vi "SL_Facade.vi"(0 "Data In":T5, 2 "Display State In":T3, 3 "Container State":T4) -> (6 "Data Out":T5, 7 "Display State Out":T3, 8 "Action":T2)   [LabVIEW 2019, in "SL_XControl.xctl"]
uses:
  SL_XControl.xctl
  SL_Data.ctl
  <vilib>/_xctls/Container State.ctl
  SL_State.ctl
  <vilib>/_xctls/Action.ctl
  <vilib>/_xctls/XControlSupport.lvlib
panel:
  out "Toggle":bool
  out "info":string
  in  "Refresh":bool
  in  "Login":bool
  in  "Edit":bool
  in  "Tag":T1
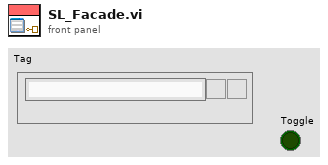
[diagram p1: front panel]
types:
  T1 = cluster{"Property":string, "Type":string, "Data":string}
  T2 = typedef "XControlSupport.lvlib/Action.ctl" = cluster{"Data Changed?":bool, "State Changed?":bool, "Action Name":string}
  T3 = typedef "SL_XControl.xctl/SL_State.ctl" = cluster{"Numeric":dbl}
  T4 = typedef "XControlSupport.lvlib/Container State.ctl" = cluster{"Indicator?":bool, "Run Mode?":bool, " Refnum":refnum<vi>}
  T5 = typedef "SL_XControl.xctl/SL_Data.ctl" = cluster{"Tag":string, "Type":string, "Data":string}
  T6 = enum8{"Enabled", "Disabled", "Disabled and Grayed Out"}
  T7 = cluster{"Name":string, "BaseURL":string, "AppKey":string, "Headers":string[], "Timeout":i32}
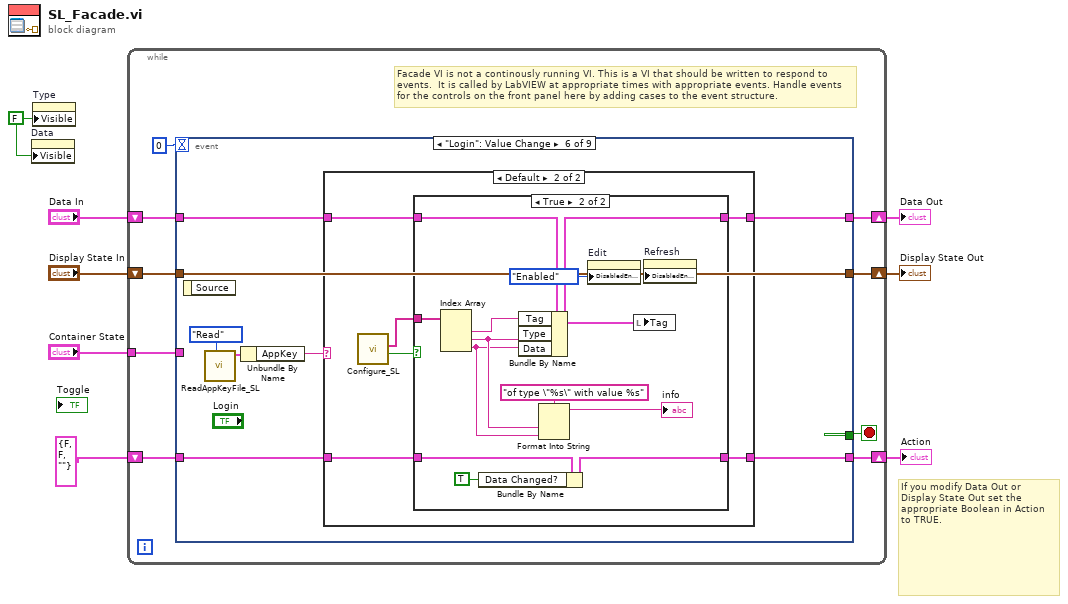
[diagram p0: block diagram]
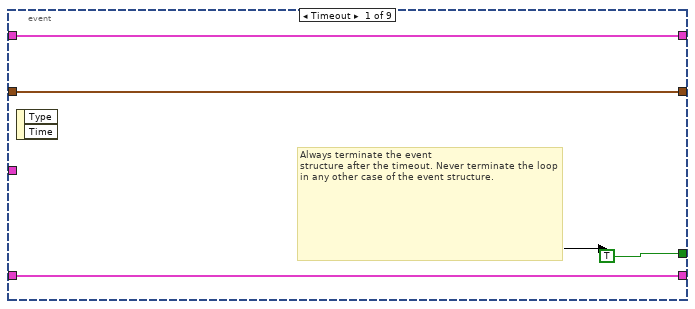
[diagram p2: hidden frame]
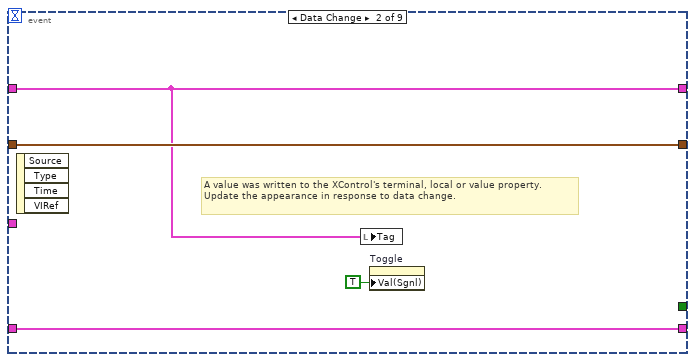
[diagram p3: hidden frame]
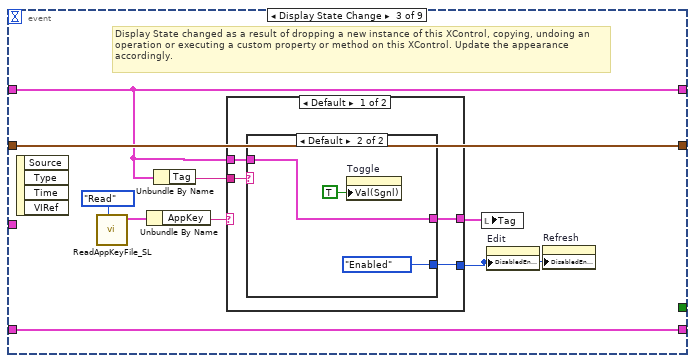
[diagram p4: hidden frame]
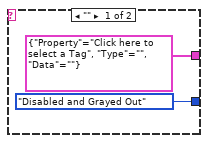
[diagram p5: hidden frame]
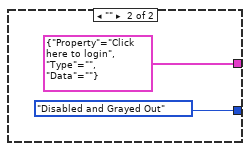
[diagram p6: hidden frame]
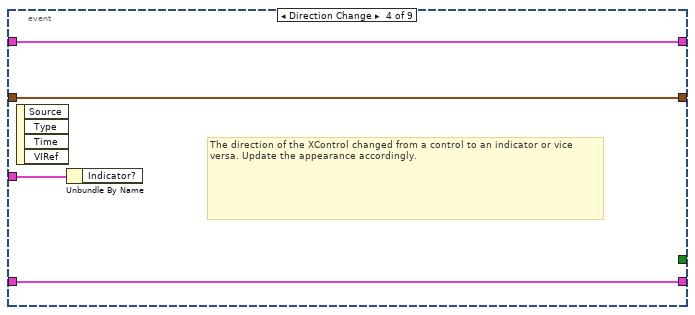
[diagram p7: hidden frame]
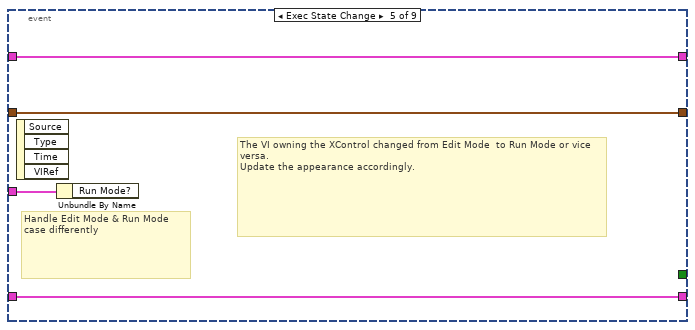
[diagram p8: hidden frame]
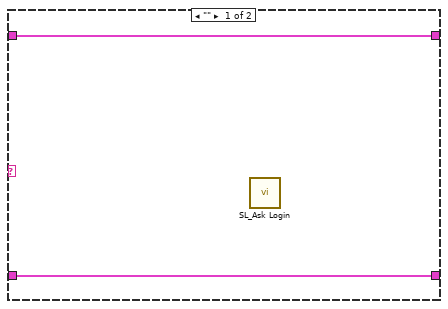
[diagram p9: hidden frame]
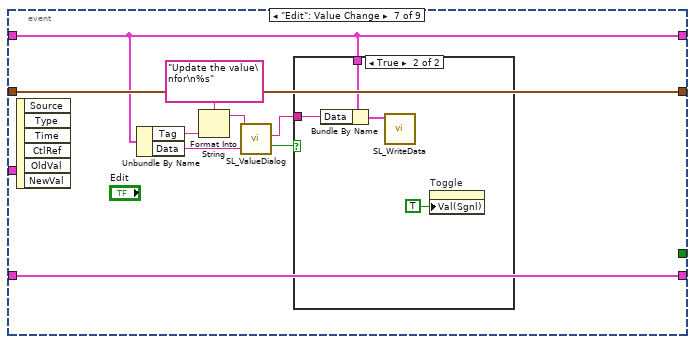
[diagram p11: hidden frame]
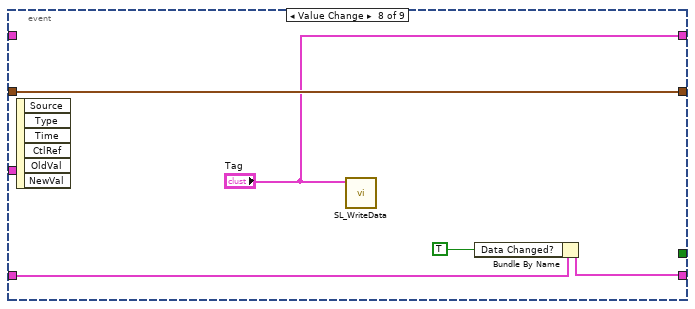
[diagram p13: hidden frame]
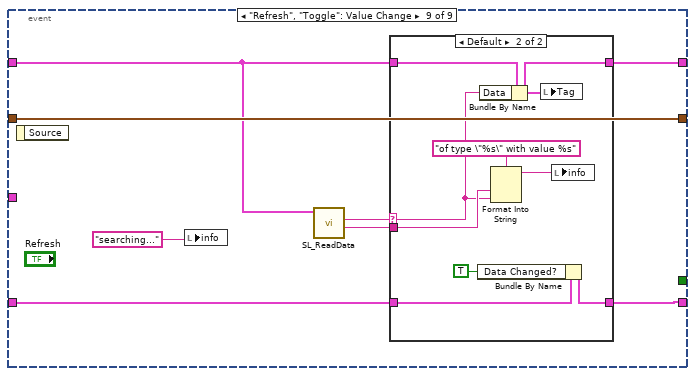
[diagram p14: hidden frame]
diagram:
  w1 = FALSE ("Visible")
  # "If you modify Data Out or\nDisplay State Out set the\nappropriate Boolean in Action\nto TRUE."
  n1 = property on="Data" class="Str"("Visible"=w1) -> ()  [unwired: 2 in, 2 out]
  n2 = property on="Type" class="Str"("Visible"=w1) -> ()  [unwired: 2 in, 2 out]
  n3 = while {
    shift-right: [w16] -> w5
    shift-left: "Display State In" -> [w17]
    tunnel: "Container State" -> [w13]
    shift-right: [w11] -> w8
    shift-left: "Data In" -> [w12]
    shift-right: [w9] -> w3
    shift-left: T2 {"Data Changed?"=FALSE, "State Changed?"=FALSE, "Action Name"=""} ("Action") -> [w10]
    stop <- w15 stop-if-true
    # "Facade VI is not a continously running VI. This is a VI that should be written to respond to events.  It is called by LabVIEW at appropriate times with appropriate events. Handle events for the controls on the front panel here by adding cases to the event structure."
    n4 = event shown="[5] \"Login\": Value Change" {
      selector: _ -> [_ _ _ _ _ _ _ _ _]
      dyn-events: _ -> [_ _ _ _ _ _ _ _ _]
      timeout: 0 -> [_ _ _ _ _ _ _ _ _]
      tunnel: w17 -> [w19 w25 w34 w48 w52 w61 w92 w101 w109]
      tunnel: [w19 w25 w34 w48 w52 w61 w92 w101 w109] -> w16
      tunnel: [TRUE _ _ _ _ _ _ _ _] -> w15
      tunnel: w13 -> [_ _ _ w49 w53 _ _ _ _]
      tunnel: w12 -> [w18 w22 w26 w47 w51 w58 w88 _ w105]
      tunnel: [w18 w22 w26 w47 w51 w57 w88 "Tag" w108] -> w11
      tunnel: [w20 w24 w33 w46 w50 w59 w91 w98 w106] -> w9
      tunnel: w10 -> [w20 w24 w33 w46 w50 w60 w91 w99 w107]
      event Timeout {
        # "Always terminate the event\nstructure after the timeout. Never terminate the loop in any other case of the event structure."
        n5 = event-data() -> ()  [unwired: 1 in, 2 out]
      }
      event Data Change {
        # "A value was written to the XControl's terminal, local or value property.\nUpdate the appearance in response to data change."
        n6 = event-data() -> ()  [unwired: 1 in, 4 out]
        n7 = local write "Tag"(w22) -> ()
        n8 = property on="Toggle" class="Bool (strict)"("Val(Sgnl)"=TRUE ("Value (Signaling)")) -> ()  [unwired: 2 in, 2 out]
      }
      event Display State Change {
        # "Display State changed as a result of dropping a new instance of this XControl, copying, undoing an operation or executing a custom property or method on this XControl. Update the appearance accordingly."
        n9 = event-data() -> ()  [unwired: 1 in, 4 out]
        n10 = call "ReadAppKeyFile_SL.vi"("Task"=enum16{"Read", "Write"}."Read") -> ("Device Out"=w32:T7)  [unwired: 8 in, 2 out]
        n11 = Unbundle By Name(w32) -> ("AppKey"=w31:string)
        n12 = Unbundle By Name(w26) -> ("Tag"=w27:string)
        n13 = case shown="Default" w31 {
          tunnel: [w38 T1 {"Property"="Click here to login", "Type"="", "Data"=""} ("Tag")] -> w30
          tunnel: [w37 T6."Disabled and Grayed Out" ("Disabled")] -> w29
          tunnel: w27 -> [w36 _]
          tunnel: w26 -> [w35 _]
          frame Default {
            n14 = case shown="Default" w36 {
              tunnel: [T1 {"Property"="Click here to select a Tag", "Type"="", "Data"=""} ("Tag") w42] -> w38
              tunnel: [T6."Disabled and Grayed Out" ("Disabled") T6."Enabled" ("Disabled")] -> w37
              tunnel: w35 -> [_ w42]
              frame "" {
              }
              frame Default {
                n15 = property on="Toggle" class="Bool (strict)"("Val(Sgnl)"=TRUE ("Value (Signaling)")) -> ()  [unwired: 2 in, 2 out]
              }
            }
          }
          frame "" {
          }
        }
        n16 = local write "Tag"(w30) -> ()
        n17 = property on="Edit" class="Bool"("DisabledEnum"=w29) -> ()  [unwired: 2 in, 2 out]
        n18 = property on="Refresh" class="Bool"("DisabledEnum"=w29) -> ()  [unwired: 2 in, 2 out]
      }
      event Direction Change {
        # "The direction of the XControl changed from a control to an indicator or vice versa. Update the appearance accordingly."
        n19 = event-data() -> ()  [unwired: 1 in, 4 out]
        n20 = Unbundle By Name(w49) -> ()  [unwired: 1 out]
      }
      event Exec State Change {
        # "The VI owning the XControl changed from Edit Mode  to Run Mode or vice versa.\nUpdate the appearance accordingly."
        # "Handle Edit Mode & Run Mode\ncase differently"
        n21 = event-data() -> ()  [unwired: 1 in, 4 out]
        n22 = Unbundle By Name(w53) -> ()  [unwired: 1 out]
      }
      event "Login": Value Change {
        n23 = event-data() -> ()  [unwired: 1 in, 1 out]
        n24 = call "ReadAppKeyFile_SL.vi"("Task"=enum16{"Read", "Write"}."Read") -> ("Device Out"=w56:T7)  [unwired: 8 in, 2 out]
        n25 = Unbundle By Name(w56) -> ("AppKey"=w54:string)
        n26 = case shown="Default" w54 {
          tunnel: w60 -> [w62 w69]
          tunnel: [w62 w68] -> w59
          tunnel: w58 -> [w63 w67]
          tunnel: [w63 w66] -> w57
          frame "" {
            n27 = call "SL_Ask Login.vi"() -> ()  [unwired: 10 in, 2 out]
          }
          frame Default {
            n28 = call "Configure_SL.vi"() -> ("changed?"=w65:bool, "Property"=w64:string[])  [unwired: 10 in]
            n29 = case shown="True" w65 {
              tunnel: w67 -> [w71 w83]
              tunnel: [w71 w78] -> w66
              tunnel: w64 -> [_ w82]
              tunnel: w69 -> [w70 w80]
              tunnel: [w70 w79] -> w68
              frame False {
              }
              frame True {
                w73 = T6."Enabled" ("Disabled")
                n30 = Index Array(array=w82) -> (element #1=w72:string, element #2=w76:string, element #3=w75:string)  [unwired: 3 in]
                n31 = Bundle By Name(cluster=w80, "Data Changed?"=TRUE) -> (w79:T2)
                n32 = Bundle By Name(cluster=w83, "Tag"=w72, "Type"=w76, "Data"=w75) -> (w78:T5)
                n33 = Format Into String(format string="of type \"%s\" with value %s", w76, w75) -> (resulting string=→"info":string)  [unwired: 2 in, 1 out]
                n34 = property on="Edit" class="Bool"("DisabledEnum"=w73) -> ()  [unwired: 2 in, 2 out]
                n35 = local write "Tag"(w78) -> ()
                n36 = property on="Refresh" class="Bool"("DisabledEnum"=w73) -> ()  [unwired: 2 in, 2 out]
              }
            }
          }
        }
      }
      event "Edit": Value Change {
        n37 = event-data() -> ()  [unwired: 1 in, 6 out]
        n38 = Unbundle By Name(w88) -> ("Tag"=w85:string, "Data"=w90:string)
        n39 = Format Into String(format string="Update the value\nfor\n%s", w85) -> (resulting string=w84:string)  [unwired: 2 in, 1 out]
        n40 = call "SL_ValueDialog.vi"("Value"=w90, "Title"=w84) -> ("replace?"=w89:bool, "Value out"=w87:string)  [unwired: 8 in]
        n41 = case shown="True" w89 {
          tunnel: w88 -> [_ w96]
          tunnel: w87 -> [_ w95]
          frame False {
          }
          frame True {
            n42 = Bundle By Name(cluster=w96, "Data"=w95) -> (w94:T5)
            n43 = call "SL_WriteData.vi"("Tag"=w94) -> ()  [unwired: 11 in]
            n44 = property on="Toggle" class="Bool (strict)"("Val(Sgnl)"=TRUE ("Value (Signaling)")) -> ()  [unwired: 2 in, 2 out]
          }
        }
      }
      event "Tag.Data": Value Change {
        n45 = event-data() -> ()  [unwired: 1 in, 6 out]
        n46 = call "SL_WriteData.vi"("Tag"="Tag") -> ()  [unwired: 11 in]
        n47 = Bundle By Name(cluster=w99, "Data Changed?"=TRUE) -> (w98:T2)
      }
      event "Refresh", "Toggle": Value Change {
        n48 = event-data() -> ()  [unwired: 1 in, 1 out]
        n49 = local write "info"("searching..." ("info")) -> ()
        n50 = call "SL_ReadData.vi"("Tag"=w105) -> ("type"=w103:string, "value"=w104:string)  [unwired: 9 in]
        n51 = case shown="Default" w104 {
          selector: w104 -> [_ w114]
          tunnel: w105 -> [w111 w120]
          tunnel: [w111 w116] -> w108
          tunnel: w107 -> [w110 w119]
          tunnel: [w110 w118] -> w106
          tunnel: w103 -> [_ w115]
          frame "" {
          }
          frame Default {
            n52 = Bundle By Name(cluster=w119, "Data Changed?"=TRUE) -> (w118:T2)
            n53 = Bundle By Name(cluster=w120, "Data"=w114) -> (w116:T5)
            n54 = Format Into String(format string="of type \"%s\" with value %s", w115, w114) -> (resulting string=w112:string)  [unwired: 2 in, 1 out]
            n55 = local write "Tag"(w116) -> ()
            n56 = local write "info"(w112) -> ()
          }
        }
      }
    }
  }
  "Display State Out" <- w5
  "Data Out" <- w8
  "Action" <- w3
